vi "showCursorTime.vi"(6 "Cursor Properties":T1={"Horizontal Line?"=TRUE, "Vertical Line?"=TRUE, "Timestamp"=enum."at BOTTOM", "time format (%H:%M:%S)"="%H:%M:%S", "size"=2, "font"={"Font Name"="Arial", "Size"=16, "Strikeout?"=FALSE, "Italic?"=FALSE, "Underline?"=FALSE, "Outline?"=FALSE, "Shadow"=FALSE, "Bold?"=FALSE}, "alignment(left, top)"={"Horizontal"=enum."center", "Vertical"=enum."center"}, "TextFormat"="%3$s\\n%2$.2f"} {"size" min=1 max=50}, 7 "Picture in":picture, 8 "error in (no error)":errorcluster, 9 "XY Values":cluster{"X":dbl, "X":dbl}, 10 "origin":cluster{"x":i16, "y":i16}, 11 "QControl_Graph in":refnum<class "QControl_Graph.lvclass">) -> (0 "error out":errorcluster, 3 "QControl_Graph out":refnum<class "QControl_Graph.lvclass">, 5 "Picture out":picture)   [LabVIEW 2017, in "QControl_Graph.lvclass"]
uses:
  QControl_Graph.lvclass
  C:/Program Files (x86)/National Instruments/LabVIEW 2017/vi.lib/QSI/QControls/QControl Classes/GraphChart/GraphChart.lvclass
  Cursor Properties.ctl
  Font.ctl
  Alignment.ctl
  Alignment.Horizontal.ctl
  Alignment.Vertical.ctl
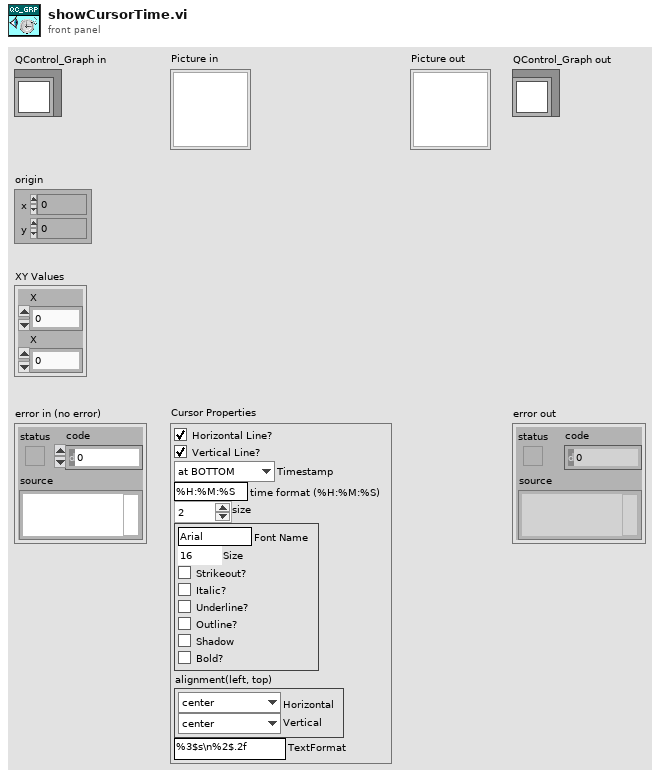
[diagram p1: front panel]
types:
  T1 = typedef "QControl_Graph.lvclass/Cursor Properties.ctl" = cluster{"Horizontal Line?":bool, "Vertical Line?":bool, "Timestamp":enum16{"at TOP", "at BOTTOM", "none"}, "time format (%H:%M:%S)":string, "size":i16, "font":T2, "alignment(left, top)":T3, "TextFormat":string}
  T2 = typedef "QControl_Graph.lvclass/Font.ctl" = cluster{"Font Name":string, "Size":i16, "Strikeout?":bool, "Italic?":bool, "Underline?":bool, "Outline?":bool, "Shadow":bool, "Bold?":bool}
  T3 = typedef "QControl_Graph.lvclass/Alignment.ctl" = cluster{"Horizontal":T4, "Vertical":T5}
  T4 = typedef "QControl_Graph.lvclass/Alignment.Horizontal.ctl" = enum16{"left", "center", "right"}
  T5 = typedef "QControl_Graph.lvclass/Alignment.Vertical.ctl" = enum16{"top", "center", "bottom"}
  T6 = cluster{"horizontal":enum16{"left", "center", "right"}, "vertical":enum16{"top", "center", "bottom"}}
  T7 = enum16{"User-specified Font", "Application Font", "System Font", "Dialog Font"}
  T8 = typedef "LVRectTypeDef.ctl" = cluster{"Left":i16, "Top":i16, "Right":i16, "Bottom":i16}
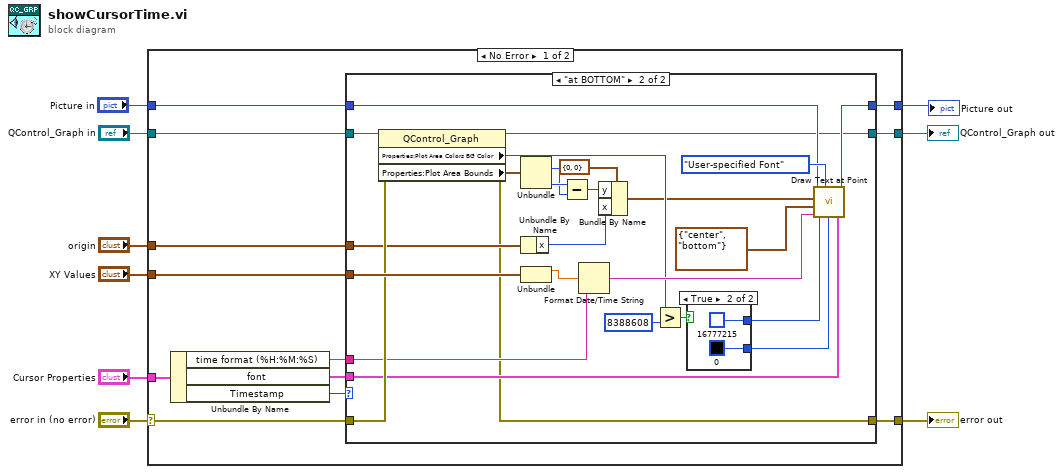
[diagram p0: block diagram]
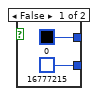
[diagram p3: hidden frame]
diagram:
  n1 = case shown="No Error" "error in (no error)" {
    selector: "error in (no error)" -> [w17 w57]
    tunnel: [w16 w57] -> w8
    tunnel: [w20 w56] -> w6
    tunnel: "QControl_Graph in" -> [w21 w56]
    tunnel: "Cursor Properties" -> [w19 _]
    tunnel: "origin" -> [w13 _]
    tunnel: "XY Values" -> [w18 _]
    tunnel: "Picture in" -> [w11 w55]
    tunnel: [w10 w55] -> w1
    frame No Error {
      n2 = Unbundle By Name(w19) -> ("time format (%H:%M:%S)"=w15:string, "font"=w14:T2, "Timestamp"=w12:enum16{"at TOP", "at BOTTOM", "none"})
      n3 = case shown="\"at BOTTOM\"" w12 {
        tunnel: w21 -> [w23 w50]
        tunnel: [w23 w27] -> w20
        tunnel: w18 -> [_ w49]
        tunnel: w17 -> [w24 w48]
        tunnel: [w24 w26] -> w16
        tunnel: w15 -> [_ w46]
        tunnel: w14 -> [_ w41]
        tunnel: w13 -> [_ w37]
        tunnel: w11 -> [w22 w29]
        tunnel: [w22 w28] -> w10
        frame "at TOP", Default {
        }
        frame "at BOTTOM" {
          n4 = property class="QControl_Graph"(reference=w50, error in=w48) -> (reference out=w27:refnum<class "QControl_Graph.lvclass">, error out=w26:errorcluster, "Properties:Plot Area Colors BG Color"=w44:u32, "Properties:Plot Area Bounds"=w36:T8)
          n5 = Unbundle(w36) -> ("Top"=w34:i16, "Bottom"=w35:i16)  [unwired: 2 out]
          n6 = Unbundle By Name(w37) -> ("x"=w30:i16)
          n7 = Unbundle(w49) -> ("X"=w25:dbl)  [unwired: 1 out]
          n8 = Subtract(x=w35, y=w34) -> (x-y=w31:i16)
          n9 = Format Date/Time String(time format string (%c)=w46, seconds (now)=w25) -> (date/time string=w45:string)  [unwired: 1 in]
          n10 = Bundle By Name(cluster=cluster{"x":i16, "y":i16} {"x"=0, "y"=0} ("origin"), "y"=w31, "x"=w30) -> (w32:cluster{"x":i16, "y":i16})
          n11 = Greater?(x=w44, y=u32 8388608) -> (0:w42:bool)
          n12 = case shown="True" w42 {
            tunnel: [u32 0 u32 16777215] -> w40
            tunnel: [u32 16777215 u32 0] -> w39
            frame False {
            }
            frame True {
            }
          }
          n13 = call <vilib>:"Draw Text at Point.vi"("BG color(transparent)"=w39, "[user-specified font]"=w41, "text color(black)"=w40, "desired font(Application)"=T7."User-specified Font", "text"=w45, "alignment(left, top)"=T6 {"horizontal"=enum."center", "vertical"=enum."bottom"}, "origin"=w32, "picture"=w29) -> ("new picture"=w28:picture)  [unwired: 2 in, 1 out]
        }
      }
    }
    frame Error {
    }
  }
  "error out" <- w8
  "QControl_Graph out" <- w6
  "Picture out" <- w1
